vi "determine more warnings.vi"() -> ()   [LabVIEW 2014]
panel:
  in  "max wind speed":dbl
  in  "current wind speed":dbl
  out "warning?":bool
  out "warning text":string
  in  "min temp":dbl
  in  "max temp":dbl
  in  "current temp":dbl
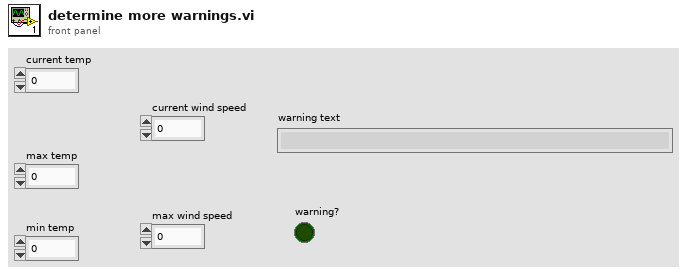
[diagram p1: front panel]
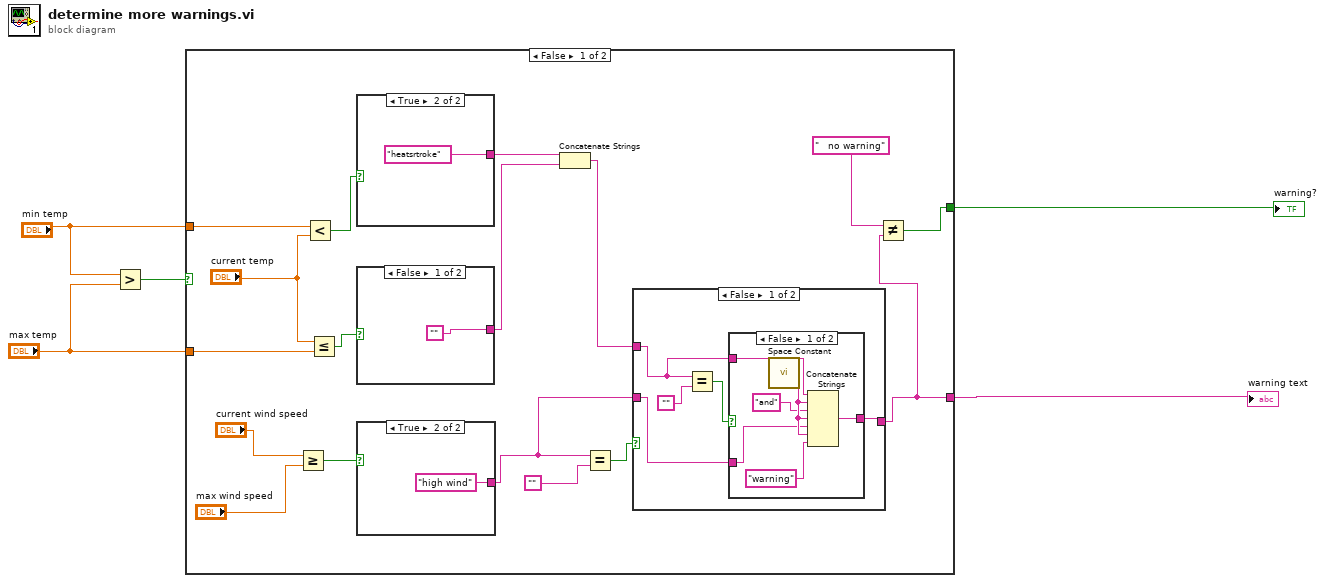
[diagram p0: block diagram]
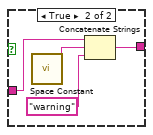
[diagram p2: hidden frame]
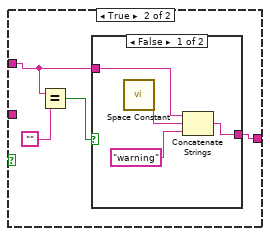
[diagram p3: hidden frame]
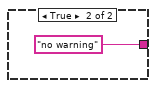
[diagram p4: hidden frame]
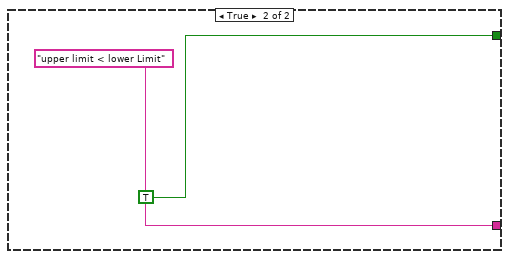
[diagram p8: hidden frame]
diagram:
  n1 = Greater?(x="min temp", y="max temp") -> (0:w3:bool)
  n2 = case shown="False" w3 {
    tunnel: "min temp" -> [w22 _]
    tunnel: "max temp" -> [w21 _]
    tunnel: [w7 "upper limit < lower Limit"] -> w2
    tunnel: [w8 TRUE] -> w1
    frame False {
      n3 = Greater Or Equal?(x="current wind speed", y="max wind speed") -> (x >= y?=w13:bool)
      n4 = Less?(x=w22, y="current temp") -> (x < y?=w18:bool)
      n5 = Less Or Equal?(x="current temp", y=w21) -> (x <= y?=w19:bool)
      n6 = case shown="True" w18 {
        tunnel: [_ "heatsrtroke"] -> w10
        frame False {
        }
        frame True {
        }
      }
      n7 = case shown="False" w19 {
        tunnel: ["" _] -> w11
        frame False {
        }
        frame True {
        }
      }
      n8 = case shown="True" w13 {
        tunnel: [_ "high wind"] -> w12
        frame False {
        }
        frame True {
        }
      }
      n9 = Concatenate Strings(w10, w11) -> (w9:string)
      n10 = Equal?(x=w12, y="") -> (x = y?=w16:bool)
      n11 = case shown="False" w16 {
        tunnel: w12 -> [w24 _]
        tunnel: w9 -> [w26 w39]
        tunnel: [w23 w38] -> w7
        frame False {
          n12 = Equal?(x=w26, y="") -> (x = y?=w25:bool)
          n13 = case shown="False" w25 {
            tunnel: w26 -> [w28 _]
            tunnel: w24 -> [w31 w36]
            tunnel: [w30 w37] -> w23
            frame False {
              n14 = call <vilib>:"Space Constant.vi"() -> ("String"=w33:string)
              n15 = Concatenate Strings(w28, w33, "and" ("string"), w33, w31, w33, "warning" ("string")) -> (w30:string)
            }
            frame True {
              n16 = call <vilib>:"Space Constant.vi"() -> ("String"=w35:string)
              n17 = Concatenate Strings(w36, w35, "warning" ("string")) -> (w37:string)
            }
          }
        }
        frame True {
          n18 = Equal?(x=w39, y="") -> (x = y?=w41:bool)
          n19 = case shown="False" w41 {
            tunnel: w39 -> [w43 _]
            tunnel: [w45 "no warning"] -> w38
            frame False {
              n20 = call <vilib>:"Space Constant.vi"() -> ("String"=w44:string)
              n21 = Concatenate Strings(w43, w44, "warning" ("string")) -> (w45:string)
            }
            frame True {
            }
          }
        }
      }
      n22 = Not Equal?(x="   no warning", y=w7) -> (x != y?=w8:bool)
    }
    frame True {
    }
  }
  "warning text" <- w2
  "warning?" <- w1
